vi "Untitled 1 (SubVI).vi"(11 "Numeric":i32) -> ()   [LabVIEW 2016]
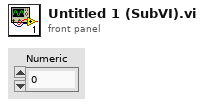
[diagram p1: front panel]
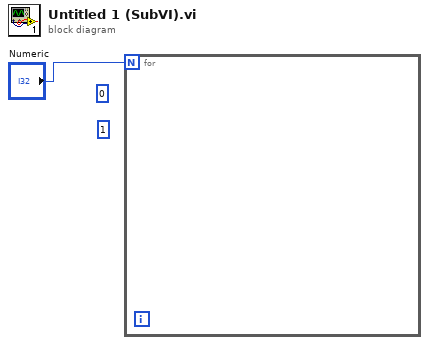
[diagram p0: block diagram]
diagram:
  (unwired) 1
  (unwired) 0
  n1 = for {
    N: "Numeric" -> [_]
  }
